vi "FormClose.vi"(8 "エラー入力（エラーなし）":errorcluster, 11 "VI入力":refnum<vi>) -> (0 "エラー出力":errorcluster)   [LabVIEW 2014]
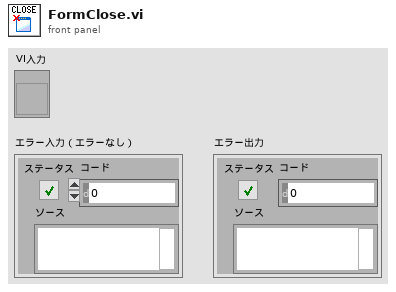
[diagram p1: front panel]
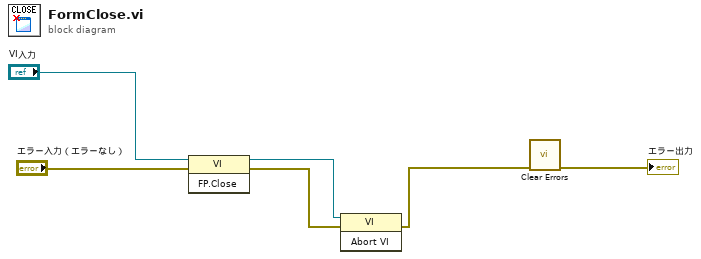
[diagram p0: block diagram]
diagram:
  n1 = invoke class="VI" method="FP.Close"(reference="VI入力", error in="エラー入力（エラーなし）") -> (reference out=w4:refnum<vi>, error out=w3:errorcluster)  [unwired: 1 in, 1 out]
  n2 = invoke class="VI" method="Abort VI"(reference=w4, error in=w3) -> (error out=w2:errorcluster)  [unwired: 1 in, 2 out]
  n3 = call <vilib>:"Clear Errors.vi"("error in (no error)"=w2) -> ("error out"=→"エラー出力":errorcluster)  [unwired: 5 in, 1 out]
